vi "Labview Sound Receive Tester.vi"() -> ()   [LabVIEW 2025]
panel:
  out "appended path":path
  out "error out":errorcluster
  out "return value":string
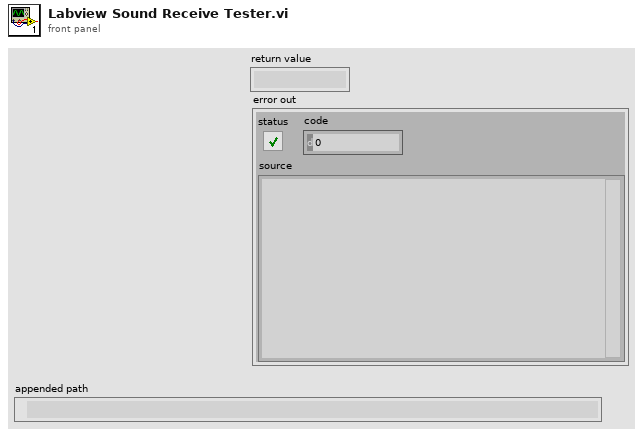
[diagram p1: front panel]
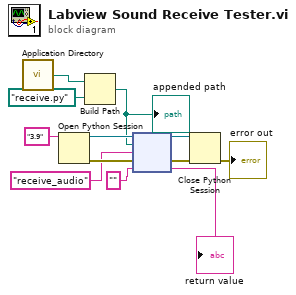
[diagram p0: block diagram]
diagram:
  n1 = call <vilib>:"Application Directory.vi"() -> ("Application Directory"=w6:path)
  n2 = Open Python Session(python version="3.9" ("Python version")) -> (session out=w12:refnum<k35>, error out=w11:errorcluster)  [unwired: 2 in]
  n3 = Build Path(base path=w6, name or relative path=path "receive.py") -> (appended path=w4:path)
  "appended path" <- w4
  n4 = node(w12, w4, "receive_audio" ("function name"), w11, "") -> (w9:refnum<k35>, w10:errorcluster, →"return value":string)  [unwired: 2 out]
  n5 = Close Python Session(session in=w9, error in=w10) -> (11:→"error out":errorcluster)
